vi "Solar Example.vi"(10 "solartracker":refnum<visa-resource-name>) -> ()   [LabVIEW 2026]
uses:
  <vilib>/Instr/_visa.llb/VISA Configure Serial Port (Instr).vi
panel:
  out "error out":errorcluster
  out "read buffer":string
  in  "stop":bool
  out "Waveform Chart":dbl(graph)
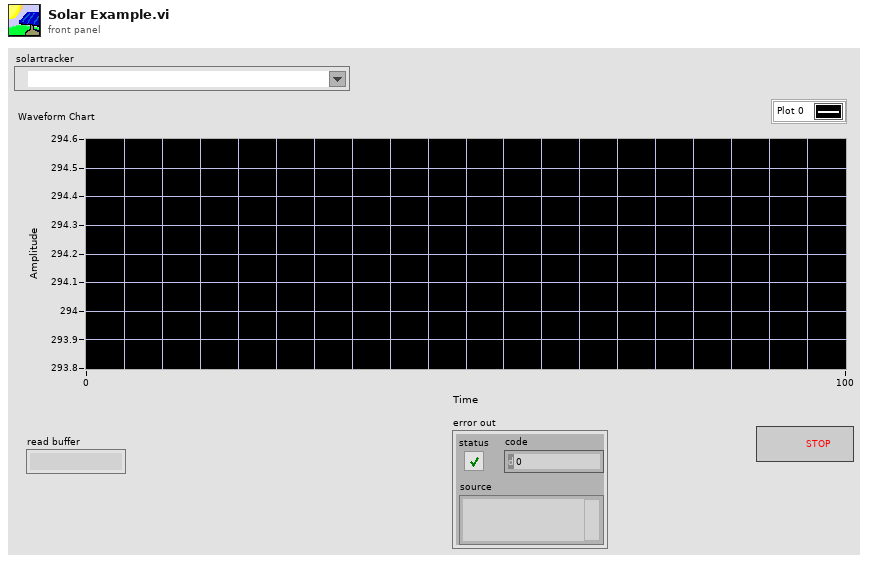
[diagram p1: front panel]
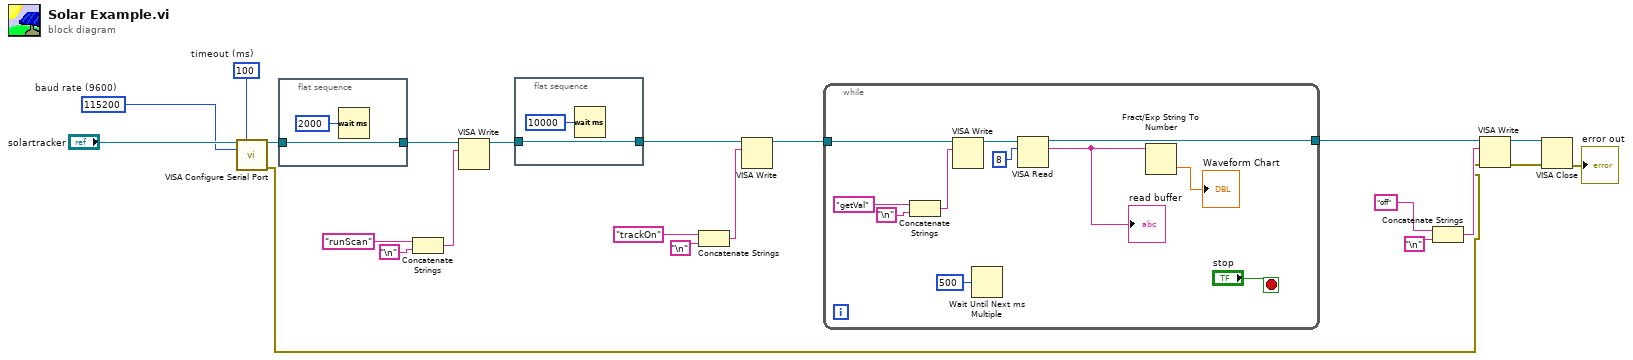
[diagram p0: block diagram]
diagram:
  w5 = u32 115200  # baud rate (9600)
  w4 = u32 100  # timeout (ms)
  n1 = call-poly "VISA Configure Serial Port"("VISA resource name"="solartracker", "timeout (10sec)"=w4, "baud rate (9600)"=w5) -> ("VISA resource name out"=w8:refnum<visa-resource-name>, "error out"=w3:errorcluster)  [unwired: 11 in]
  n2 = flat-sequence {
    tunnel: w8 -> [w23]
    tunnel: [w23] -> w7
    frame #0 {
      n3 = Wait (ms)(milliseconds to wait=u32 2000) -> ()  [unwired: 1 out]
    }
  }
  n4 = Concatenate Strings("runScan" ("string"), "\n") -> (w22:string)
  n5 = VISA Write(VISA resource name=w7, write buffer=w22) -> (VISA resource name out=w19:refnum<visa-resource-name>)  [unwired: 1 in, 2 out]
  n6 = flat-sequence {
    tunnel: w19 -> [w25]
    tunnel: [w25] -> w16
    frame #0 {
      n7 = Wait (ms)(milliseconds to wait=u32 10000) -> ()  [unwired: 1 out]
    }
  }
  n8 = Concatenate Strings("trackOn" ("string"), "\n") -> (w15:string)
  n9 = VISA Write(VISA resource name=w16, write buffer=w15) -> (VISA resource name out=w14:refnum<visa-resource-name>)  [unwired: 1 in, 2 out]
  n10 = while {
    tunnel: w14 -> [w35]
    tunnel: [w29] -> w11
    stop <- "stop" stop-if-true
    n11 = Concatenate Strings("getVal" ("string"), "\n") -> (w34:string)
    n12 = VISA Write(VISA resource name=w35, write buffer=w34) -> (VISA resource name out=w33:refnum<visa-resource-name>)  [unwired: 1 in, 2 out]
    n13 = Wait Until Next ms Multiple(millisecond multiple=u32 500) -> ()  [unwired: 1 out]
    n14 = VISA Read(VISA resource name=w33, byte count=u32 8) -> (VISA resource name out=w29:refnum<visa-resource-name>, read buffer=w27:string)  [unwired: 1 in, 2 out]
    "read buffer" <- w27
    n15 = Fract/Exp String To Number(string=w27) -> (number=→"Waveform Chart":dbl)  [unwired: 3 in, 1 out]
  }
  n16 = Concatenate Strings("off" ("string"), "\n") -> (w10:string)
  n17 = VISA Write(VISA resource name=w11, write buffer=w10, error in (no error)=w3) -> (VISA resource name out=w9:refnum<visa-resource-name>, error out=w2:errorcluster)  [unwired: 1 out]
  n18 = VISA Close(VISA resource name=w9, error in (no error)=w2) -> (error out=→"error out":errorcluster)
